vi "Test sort.vi"(11 "Error in":errorcluster) -> (15 "Error out":errorcluster)   [LabVIEW 2020, in "BubbleSort Tests.lvlib"]
doc: "This VI validates Bubble sort"
uses:
  BubbleSort Tests.lvlib
  <vilib>/addons/_JKI Toolkits/Caraya/classes/Test Suite/Define Test Suite (JUnit Report).vi
  <vilib>/SLL Drona/APIs/Stimulus/ControlValue/SetValueAuto.vi
  <vilib>/SLL Drona/APIs/Assert/AssertControlValue/Equal.vi
  <vilib>/SLL Drona/APIs/Stimulus/VI/CloseVI.vi
  <vilib>/Utility/error.llb/Error Cluster From Error Code.vi
  <vilib>/ErrorRing/Error Ring.xnode
  <vilib>/addons/_JKI Toolkits/Caraya/classes/Test Suite/Test Suite.lvclass
  <vilib>/addons/_JKI Toolkits/Caraya/classes/Test/Test.lvclass
  <vilib>/SLL Drona/Drona.lvlib
  <vilib>/SLL Drona/APIs/Stimulus/ControlValue/ControlValue.lvlib
  <vilib>/Wiresmith Technology/G CLI/CLI Class/CLI.lvclass
  <vilib>/SLL Drona/APIs/Stimulus/VI/VI.lvlib
  <vilib>/SLL Drona/APIs/Assert/AssertControlValue/AssertControlValue.lvlib
panel:
  # "BUBBLE SORT TEST"
  # "Test Sort"
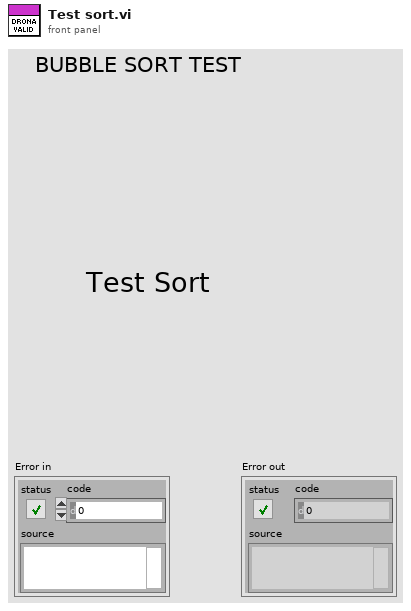
[diagram p1: front panel]
types:
  T1 = cluster{"Input Array":dbl[], "Sorting order":enum16{"Descending Order", "Ascending Order"}, "Output Array":dbl[]}[]
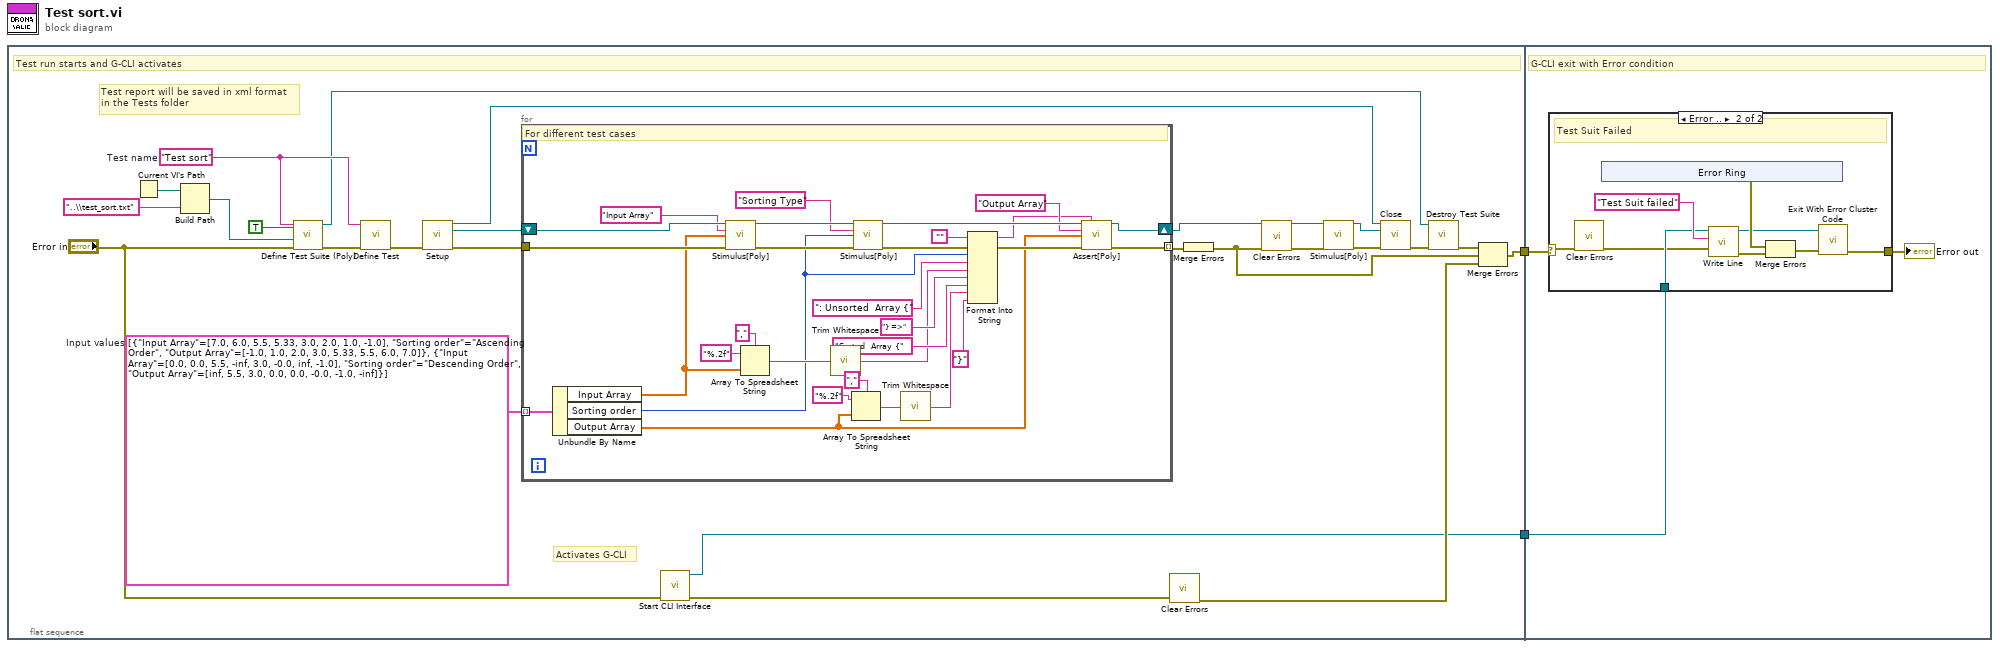
[diagram p0: block diagram]
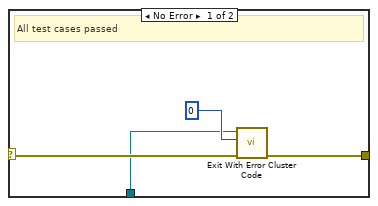
[diagram p2: hidden frame]
diagram:
  n1 = flat-sequence {
    tunnel: [w18] -> w2
    tunnel: [w15] -> w1
    tunnel: w2 -> [w60]
    tunnel: w1 -> [w58]
    frame #0 {
      w27 = T1 [{"Input Array"=[7.0, 6.0, 5.5, 5.33, 3.0, 2.0, 1.0, -1.0], "Sorting order"=enum."Ascending Order", "Output Array"=[-1.0, 1.0, 2.0, 3.0, 5.33, 5.5, 6.0, 7.0]}, {"Input Array"=[0.0, 0.0, 5.5, -inf, 3.0, -0.0, inf, -1.0], "Sorting order"=enum."Descending Order", "Output Array"=[inf, 5.5, 3.0, 0.0, 0.0, -0.0, -1.0, -inf]}]  # Input values
      w13 = "Test sort"  # Test name
      # "Test report will be saved in xml format\nin the Tests folder"
      # "Activates G-CLI"
      # "Test run starts and G-CLI activates"
      n2 = Current VI's Path() -> (path=w10:path)
      n3 = Build Path(base path=w10, name or relative path="..\\test_sort.txt") -> (appended path=w8:path)
      n4 = call-poly <vilib>:"Define Test Suite (Poly).vi"("error in (no error)"="Error in", "Report Path"=w8, "Interactive"=TRUE, "Label (VI Title)"=w13) -> ("error out"=w14:errorcluster, "Test Suite"=w5:refnum<class "Test Suite.lvclass">)  [unwired: 6 in]
      n5 = call <vilib>:"Define Test.vi"("error in (no error)"=w14, "Label (VI Title)"=w13) -> ("error out"=w26:errorcluster)  [unwired: 9 in]
      n6 = call <vilib>:"Setup.vi"("error in"=w26) -> ("Application Ref"=w23:refnum<vi>, "VI Reference Out"=w24:refnum<vi>, "error out"=w25:errorcluster)  [unwired: 12 in]
      n7 = for {
        tunnel: w27 -> [w56] mode=indexing
        shift-right: [w40] -> w21
        shift-left: w24 -> [w55]
        tunnel: w25 -> [w57]
        tunnel: [w47] -> w19 mode=indexing
        # "For different test cases"
        n8 = Unbundle By Name(w56) -> ("Input Array"=w39:dbl[], "Sorting order"=w28:enum16{"Descending Order", "Ascending Order"}, "Output Array"=w35:dbl[])
        n9 = call-poly <vilib>:"Stimulus[Poly].vi"("VI Reference In"=w55, "Control Path"="Input Array", "Value (Signaling)"=w39, "error in"=w57) -> ("VI Reference Out"=w52:refnum<vi>, "error out"=w53:errorcluster)  [unwired: 10 in]
        n10 = Array To Spreadsheet String(delimiter (Tab)=",", array=w39, 3:"%.2f" ("format string")) -> (spreadsheet string=w36:string)
        n11 = call <vilib>:"Trim Whitespace.vi"("string"=w36) -> ("trimmed string"=w31:string)  [unwired: 1 in]
        n12 = Array To Spreadsheet String(delimiter (Tab)=",", array=w35, 3:"%.2f" ("format string")) -> (spreadsheet string=w32:string)
        n13 = call-poly <vilib>:"Stimulus[Poly].vi"("VI Reference In"=w52, "Control Path"="Sorting Type", "Value (Signaling)"=w28, "error in"=w53) -> ("VI Reference Out"=w46:refnum<vi>, "error out"=w50:errorcluster)  [unwired: 10 in]
        n14 = call <vilib>:"Trim Whitespace.vi"("string"=w32) -> ("trimmed string"=w30:string)  [unwired: 1 in]
        n15 = Format Into String(initial string="", error in=w50, w28, ": Unsorted  Array {" ("Control Path"), w31, "} =>" ("Control Path"), "Sorted  Array {" ("Control Path"), w30, "}" ("input 6")) -> (resulting string=w41:string, error out=w48:errorcluster)  [unwired: 1 in]
        n16 = call-poly <vilib>:"Assert[Poly].vi"("VI Reference In"=w46, "Test Label"=w41, "Control Path"="Output Array", "Control Value"=w35, "Error In"=w48) -> ("VI Reference Out"=w40:refnum<vi>, "Error Out"=w47:errorcluster)  [unwired: 9 in]
      }
      n17 = call <vilib>:"Start CLI Interface.vi"("error in (no error)"="Error in") -> ("error out"=w16:errorcluster, "CLI out"=w15:refnum<class "CLI.lvclass">)  [unwired: 7 in, 2 out]
      n18 = call <vilib>:"Clear Errors.vi"("error in (no error)"=w16) -> ("error out"=w17:errorcluster)  [unwired: 5 in, 1 out]
      n19 = Merge Errors(w19) -> (w3:errorcluster)
      n20 = call <vilib>:"Clear Errors.vi"("error in (no error)"=w3) -> ("error out"=w4:errorcluster)  [unwired: 5 in, 1 out]
      n21 = call-poly <vilib>:"Stimulus[Poly].vi"("VI Reference In"=w21, "error in"=w4) -> ("VI Reference Out"=w20:refnum<vi>, "error out"=w22:errorcluster)  [unwired: 12 in]
      n22 = call <vilib>:"Close.vi"("Application Ref"=w23, "VI Reference"=w20, "error in"=w22) -> ("error out"=w7:errorcluster)  [unwired: 12 in]
      n23 = call-dynamic "Destroy Test Suite.vi"("error in (no error)"=w7, "Test Suite in"=w5) -> ("error out"=w6:errorcluster)  [unwired: 8 in, 1 out]
      n24 = Merge Errors(w6, w3, w17) -> (w18:errorcluster)
    }
    frame #1 {
      # "G-CLI exit with Error condition"
      n25 = case shown="Error .." w60 {
        selector: w60 -> [w64 w71]
        tunnel: [w62 w73] -> w59
        tunnel: w58 -> [w61 w70]
        frame No Error {
          # "All test cases passed"
          n26 = call <vilib>:"Exit With Error Cluster Code.vi"("error in (no error)"=w64, "No Error Code (0)"=0, "CLI in"=w61) -> ("error out"=w62:errorcluster)  [unwired: 8 in]
        }
        frame Error {
          # "Test Suit Failed"
          n27 = call <vilib>:"Clear Errors.vi"("error in (no error)"=w71) -> ("error out"=w65:errorcluster)  [unwired: 5 in, 1 out]
          n28 = xnode "Error Ring"() -> ("error out"=w68:errorcluster)
          n29 = call <vilib>:"Write Line.vi"("error in (no error)"=w65, "Text to Write"="Test Suit failed", "CLI in"=w70) -> ("error out"=w67:errorcluster, "CLI out"=w66:refnum<class "CLI.lvclass">)  [unwired: 7 in]
          n30 = Merge Errors(w68, w67) -> (w69:errorcluster)
          n31 = call <vilib>:"Exit With Error Cluster Code.vi"("error in (no error)"=w69, "CLI in"=w66) -> ("error out"=w73:errorcluster)  [unwired: 9 in]
        }
      }
      "Error out" <- w59
    }
  }
